vi "SubDeadOrAllive.vi"(11 "Array":u32[][](array[colorbox])) -> (3 "Array Dead Or Allive":u32[][](array[numeric]))   [LabVIEW 2013]
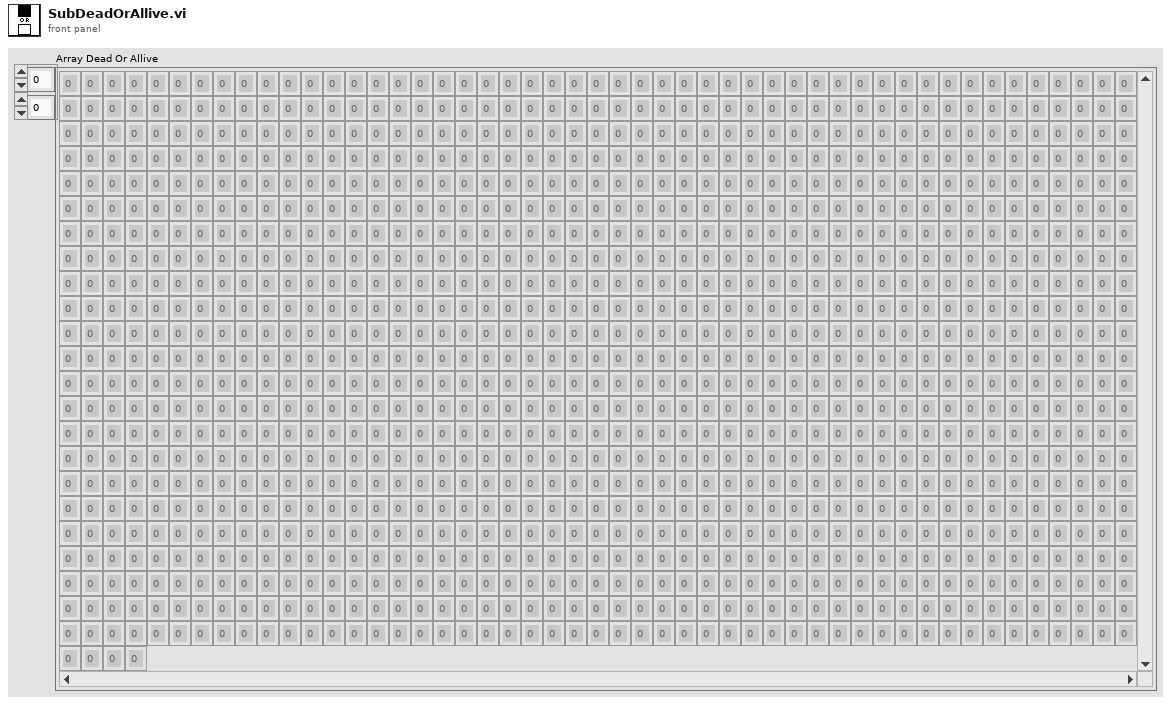
[diagram p1: front panel]
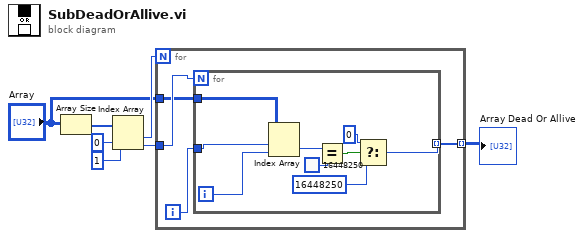
[diagram p0: block diagram]
diagram:
  n1 = Array Size(array="Array") -> (size(s)=w7:i32[])
  n2 = Index Array(array=w7, index #1=0 ("index"), index #2=1 ("index")) -> (element #1=w4:i32, element #2=w3:i32)
  n3 = for {
    N: w4 -> [_]
    tunnel: [w10] -> w1 mode=indexing
    tunnel: w3 -> [w9]
    tunnel: "Array" -> [w8]
    i -> [w11]
    n4 = for {
      N: w9 -> [_]
      tunnel: w11 -> [w20]
      tunnel: [w12] -> w10 mode=indexing
      tunnel: w8 -> [w18]
      i -> [w19]
      n5 = Index Array(array=w18, index (row)=w20, index (col)=w19) -> (element=w17:u32)
      n6 = Equal?(x=w17, y=u32 16448250) -> (x = y?=w15:bool)
      n7 = Select(t=u32 0, s=w15, f=u32 16448250 ("y")) -> (s? t:f=w12:u32)
    }
  }
  "Array Dead Or Allive" <- w1
